vi "Audio Playback.vi"(8 "error in (no error)":errorcluster, 11 "Channel in":T1) -> (0 "error out":errorcluster)   [LabVIEW 2016]
uses:
  <extravilib>/ChannelInstances/Stream-wfm(dbl)/)Channel.ctl
  <vilib>/sound2/lvsound2.llb/Sampling Mode.ctl
  <vilib>/sound2/lvsound2.llb/Sound Data Format.ctl
  <extravilib>/ChannelInstances/Stream-wfm(dbl)/Read With Abort.vi
  <extravilib>/ChannelInstances/Stream-wfm(dbl)/Endpoint.vi
  <extravilib>/ChannelInstances/Stream-wfm(dbl)/)Channel.vi
  <resource>/ChannelSupport/_ChannelSupport/WaitIfNeeded.vi
  <vilib>/sound2/lvsound2.llb/Sound Output Write (DBL Single).vi
  <extravilib>/ChannelInstances/Stream-wfm(dbl).lvlib
panel:
  out "count":i32
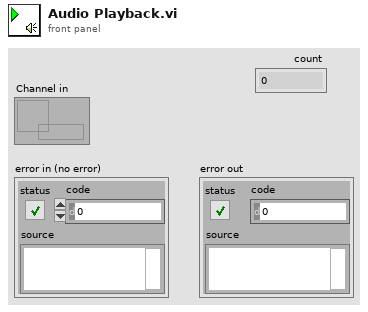
[diagram p1: front panel]
types:
  T1 = typedef "Stream-wfm(dbl).lvlib/)Channel.ctl" = refnum<queue>
  T2 = typedef "Sound Data Format.ctl" = cluster{"sample rate (S/s)":dbl, "number of channels":i32, "bits per sample":i32}
  T3 = typedef "Sampling Mode.ctl" = i32
  T4 = typedef "Sound Output Task ID.ctl" = u32
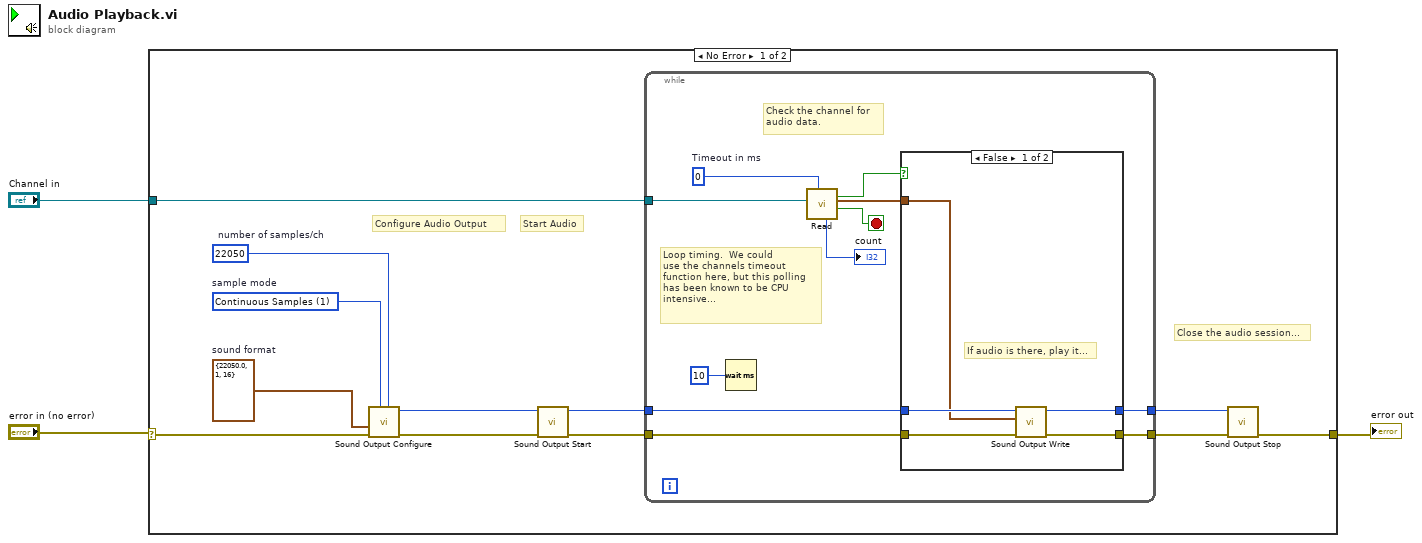
[diagram p0: block diagram]
diagram:
  n1 = case shown="No Error" "error in (no error)" {
    selector: "error in (no error)" -> [w4 w34]
    tunnel: [w15 w34] -> w3
    tunnel: "Channel in" -> [w13 _]
    frame No Error {
      w9 = 22050  # number of samples/ch
      w8 = T2 {"sample rate (S/s)"=22050.0, "number of channels"=1, "bits per sample"=16}  # sound format
      w5 = T3 1 items=["Finite Samples", "Continuous Samples"]  # sample mode
      # "Close the audio session..."
      # "Start Audio"
      # "Configure Audio Output"
      n2 = call <vilib>:"Sound Output Configure.vi"("number of samples/ch"=w9, "sample mode"=w5, "error in (no error)"=w4, "sound format"=w8) -> ("error out"=w6:errorcluster, "task ID"=w7:T4)  [unwired: 6 in]
      n3 = call <vilib>:"Sound Output Start.vi"("error in (no error)"=w6, "task ID"=w7) -> ("error out"=w11:errorcluster, "task ID out"=w10:T4)  [unwired: 8 in]
      n4 = while {
        tunnel: w10 -> [w26]
        tunnel: w11 -> [w25]
        tunnel: [w24] -> w12
        tunnel: [w23] -> w14
        tunnel: w13 -> [w19]
        stop <- w17 stop-if-true
        w20 = 0  # Timeout in ms
        # "Loop timing.  We could \nuse the channels timeout\nfunction here, but this polling\nhas been known to be CPU \nintensive..."
        # "Check the channel for\naudio data."
        n5 = Wait (ms)(milliseconds to wait=u32 10) -> ()  [unwired: 1 out]
        n6 = call <extravilib>:"Read.vi"("timeout in ms (-1)"=w20, "channel"=w19) -> ("last element?"=w17:bool, "element"=w22:waveform(dbl), "timed out?"=w21:bool, "count"=→"count":i32)  [unwired: 5 in, 1 out]
        n7 = case shown="False" w21 {
          tunnel: w26 -> [w31 w33]
          tunnel: w25 -> [w30 w32]
          tunnel: [w29 w32] -> w24
          tunnel: [w28 w33] -> w23
          tunnel: w22 -> [w27 _]
          frame False {
            # "If audio is there, play it..."
            # "If audio is there, play it..."
            n8 = call-poly <vilib>:"Sound Output Write.vi"("error in (no error)"=w30, "data"=w27, "task ID"=w31) -> ("error out"=w29:errorcluster, "task ID out"=w28:T4)  [unwired: 7 in]
          }
          frame True {
          }
        }
      }
      n9 = call <vilib>:"Sound Output Stop.vi"("error in (no error)"=w12, "task ID"=w14) -> ("error out"=w15:errorcluster)  [unwired: 8 in, 1 out]
    }
    frame Error {
    }
  }
  "error out" <- w3
